vi "Tcp Response.vi"(8 "error in (no error)":errorcluster, 10 "WSGI Response":T1, 11 "Conn in":refnum<k5>) -> (0 "error out":errorcluster, 3 "Conn out":refnum<k5>)   [LabVIEW 2021, in "HttpServer.lvlib"]
uses:
  HttpServer.lvlib
  TypeDefs/WSGI.ctl
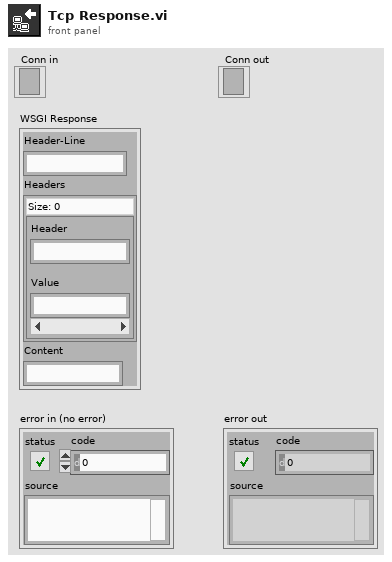
[diagram p1: front panel]
types:
  T1 = typedef "HttpServer.lvlib/WSGI.ctl" = cluster{"Header-Line":string, "Headers":map{string, string}, "Content":string}
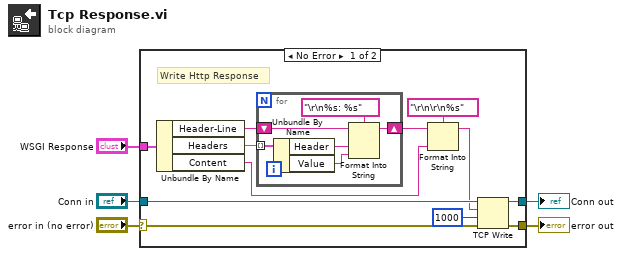
[diagram p0: block diagram]
diagram:
  n1 = case shown="No Error" "error in (no error)" {
    selector: "error in (no error)" -> [w12 w25]
    tunnel: [w17 w24] -> w1
    tunnel: [w16 w25] -> w2
    tunnel: "Conn in" -> [w15 w24]
    tunnel: "WSGI Response" -> [w6 _]
    frame No Error {
      # "Write Http Response"
      n2 = Unbundle By Name(w6) -> ("Header-Line"=w11:string, "Headers"=w7:map{string, string}, "Content"=w8:string)
      n3 = for {
        shift-right: [w18] -> w10
        shift-left: w11 -> [w23]
        tunnel: w7 -> [w22] mode=indexing
        n4 = Unbundle By Name(w22) -> ("Header"=w21:string, "Value"=w20:string)
        n5 = Format Into String(format string="\r\n%s: %s", initial string=w23, w21, w20) -> (resulting string=w18:string)  [unwired: 1 in, 1 out]
      }
      n6 = Format Into String(format string="\r\n\r\n%s", initial string=w10, w8) -> (resulting string=w14:string)  [unwired: 1 in, 1 out]
      n7 = TCP Write(connection ID=w15, data in=w14, error in (no error)=w12, 9:1000) -> (connection ID out=w17:refnum<k5>, error out=w16:errorcluster)  [unwired: 1 out]
    }
    frame Error {
    }
  }
  "error out" <- w2
  "Conn out" <- w1
